vi "Initialize Front Panel.vi"(8 "error in (no error)":errorcluster, 11 "Test Executive View in":refnum<class "Test Executive View.lvclass">) -> (0 "error out":errorcluster, 3 "Test Executive View out":refnum<class "Test Executive View.lvclass">)   [LabVIEW 2017, in "Test Executive View.lvclass"]
doc: "<License>\nCopyright © 2017 Composed Systems, LLC | All rights reserved\nwww.composed.io\n\nAuthor: Ethan Stern <ethan.stern@composed.io>\n\nThis software is provided \"AS IS\" WITHOUT WARRANTIES, either express or implied, AND IS FOR EDUCATIONAL PURPOSES ONLY.\n</License>"
uses:
  <vilib>/gpm_packages/@cs/Test-executive-builder/Example/Application/Test Executive View/Test Executive View/Test Executive View.lvclass
  C:/Program Files/National Instruments/LabVIEW 2017/vi.lib/gpm_packages/@cs/Test-executive-builder/Source/Test Executive Builder View/Test Executive Builder View/Test Executive Builder View.lvclass
  <vilib>/gpm_packages/@cs/Test-executive-builder/Source/Test Executive Builder View/Test Executive Builder View/Test Executive Builder View.lvclass/Test Executive Builder View.ctl
  <vilib>/gpm_packages/@cs/Test-executive-builder/Source/Test Executive Builder View/Test Executive Builder View/Test Executive Builder View.lvclass
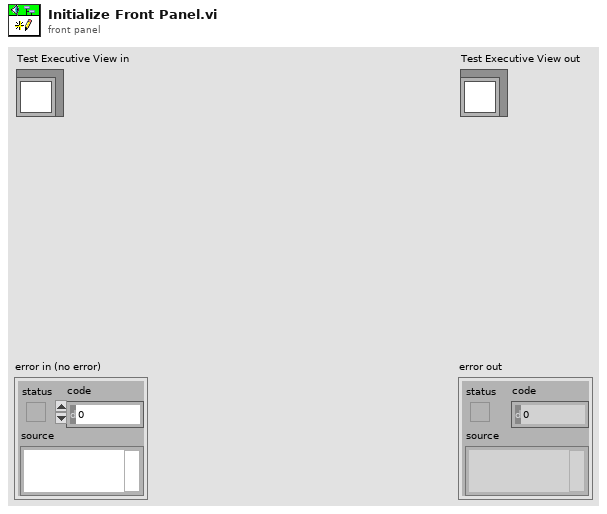
[diagram p1: front panel]
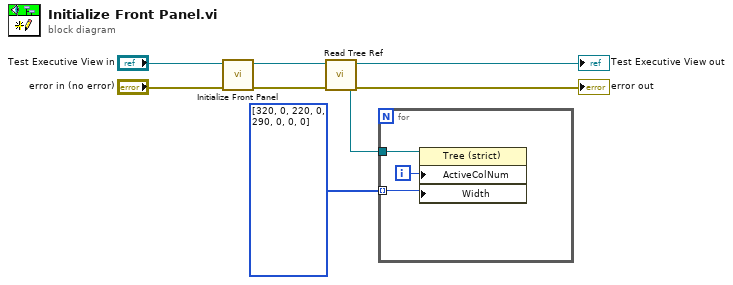
[diagram p0: block diagram]
diagram:
  n1 = call-parent "Initialize Front Panel.vi"("error in (no error)"="error in (no error)", "Test Executive Builder View in"="Test Executive View in") -> ("error out"=→"error out":errorcluster, "Test Executive Builder View out"=w4:refnum<class "Test Executive View.lvclass">)  [unwired: 8 in]
  n2 = call <vilib>:"Read Tree Ref.vi"("Test Executive Builder View in"=w4) -> ("Tree Ref"=w2:refnum<vi>, "Test Executive Builder View out"=→"Test Executive View out":refnum<class "Test Executive View.lvclass">)  [unwired: 9 in]
  n3 = for {
    tunnel: w2 -> [w10]
    tunnel: i32[] [320, 0, 220, 0, 290, 0, 0, 0] -> [w8] mode=indexing
    i -> [w9]
    n4 = property class="Tree (strict)"(reference=w10, "ActiveColNum"=w9, "Width"=w8) -> ()  [unwired: 1 in, 2 out]
  }
